vi "Shooter Wheel GetSet.vi"(9 "Enum":enum16{"Set", "Get"}(ring), 10 "Shooter Wheel DevRef In":T1={"Shooter Config reference"=refnum, "Shooter Data"={"MotorControlDevRef"={"DeviceStatus"={"status"=FALSE, "code"=0, "source"=""}, "Type"=enum."PWM", "PWM"={"PWM Channel"=enum."Invalid", "DeadBand"={"Name"="", "maxPositivePwm"=0, "minPositivePwm"=0, "centerPwm"=0, "maxNegativePwm"=0, "minNegativePwm"=0, "angularRange"=0}}, "CAN"={"Device Number"=0, "SetOutput VI Ref"=variant(enum8{"Percent VBus", "Current", "Speed", "Position", "Voltage"} enum."Percent VBus"), "GetOutput VI Ref"=variant(refnum<k1> refnum), "Enable VI Ref"=variant(dbl 12.0), "Disable VI Ref"=variant(enum8{"Percent VBus", "Speed", "Position", "Slave", "Unchanged / Invalid", "Voltage Compensation", "Current", "Motion Profile"} enum."Percent VBus"), "Data"=variant}, "Invert"=FALSE}, "CounterDevRef in"={"DevStatus"={"status"=FALSE, "code"=0, "source"=""}, "CntIndex"=enum."Ctr 0"}, "RPM Desired"=refnum, "RPM Actual"=refnum}}, 11 "DevRef":string) -> (0 "Error Out":errorcluster, 3 "Shooter Wheel DevRef Out":T1={"Shooter Config reference"=refnum, "Shooter Data"={"MotorControlDevRef"={"DeviceStatus"={"status"=FALSE, "code"=0, "source"=""}, "Type"=enum."PWM", "PWM"={"PWM Channel"=enum."Invalid", "DeadBand"={"Name"="", "maxPositivePwm"=0, "minPositivePwm"=0, "centerPwm"=0, "maxNegativePwm"=0, "minNegativePwm"=0, "angularRange"=0}}, "CAN"={"Device Number"=0, "SetOutput VI Ref"=variant(enum8{"Percent VBus", "Current", "Speed", "Position", "Voltage"} enum."Percent VBus"), "GetOutput VI Ref"=variant(refnum<k1> refnum), "Enable VI Ref"=variant(dbl 12.0), "Disable VI Ref"=variant(enum8{"Percent VBus", "Speed", "Position", "Slave", "Unchanged / Invalid", "Voltage Compensation", "Current", "Motion Profile"} enum."Percent VBus"), "Data"=variant}, "Invert"=FALSE}, "CounterDevRef in"={"DevStatus"={"status"=FALSE, "code"=0, "source"=""}, "CntIndex"=enum."Ctr 0"}, "RPM Desired"=refnum, "RPM Actual"=refnum}})   [LabVIEW 2016, in "Shooter _Wheel.lvlib"]
doc: "Help by FRC Team 836 - The RoboBees\n\nThis VI can either set or get the control parameters of a shooter wheel depending on the users command."
uses:
  <userlib>/836-Libraries/Motion_Control/Shooter_Wheel/Shooter _Wheel.lvlib
  <vilib>/Rock Robotics/SystemInterfaces/Counter/FPGA_CounterCtrSystemIndex.ctl
  <vilib>/Rock Robotics/WPI/Counter/WPI_CounterDevRef.ctl
  <vilib>/Rock Robotics/SystemInterfaces/DIO/FPGA_DIOPWMChannel.ctl
  <vilib>/Rock Robotics/WPI/PWM/WPI_PWMDeadband.ctl
  <vilib>/Rock Robotics/WPI/MotorControl/WPI_MotorControlDeviceRef.ctl
  <userlib>/836-Libraries/Motion_Control/Shooter_Wheel/ShooterData.ctl
  <userlib>/836-Libraries/Motion_Control/Shooter_Wheel/ShooterConfig.ctl
  <userlib>/836-Libraries/Motion_Control/Shooter_Wheel/ShooterControl.ctl
  <vilib>/Rock Robotics/WPI/MotorControl/WPI_MotorControlType.ctl
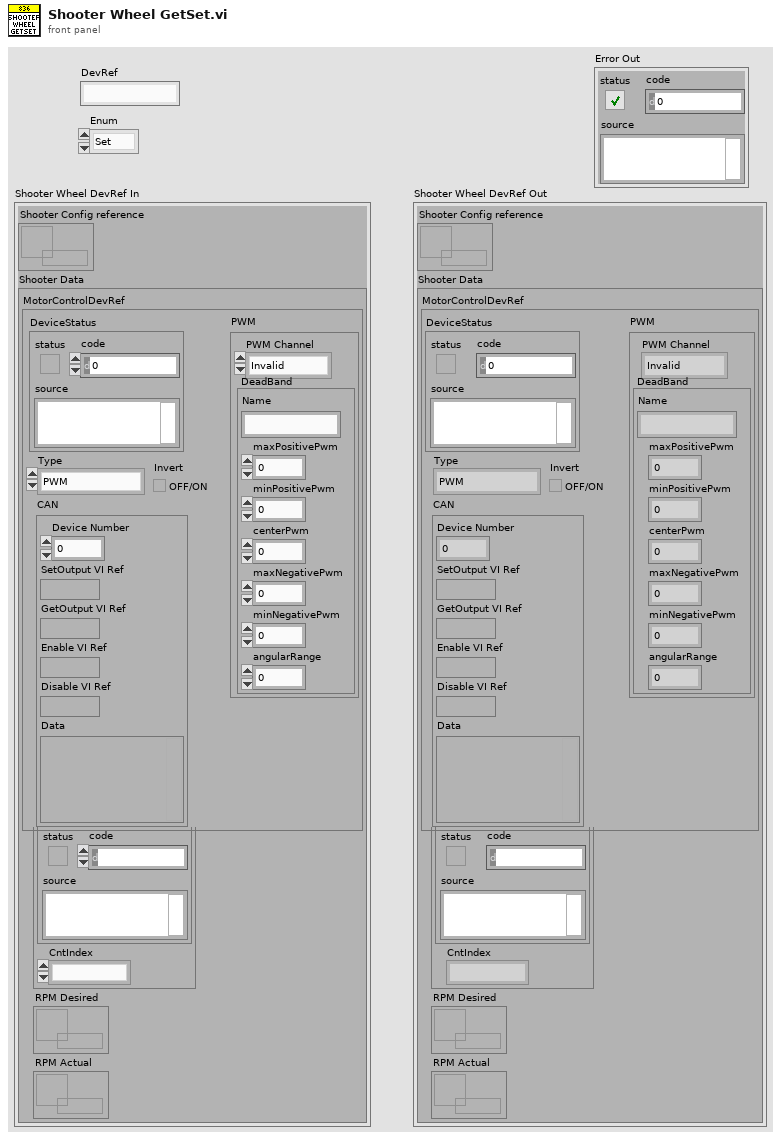
[diagram p1: front panel]
types:
  T1 = typedef "Shooter Wheel.lvlib/ShooterControl.ctl" = cluster{"Shooter Config reference":refnum<data-value>, "Shooter Data":T2}
  T2 = typedef "Shooter Wheel.lvlib/ShooterData.ctl" = cluster{"MotorControlDevRef":T3, "CounterDevRef in":T7, "RPM Desired":refnum<k33>, "RPM Actual":refnum<k33>}
  T3 = typedef "WPI_MotorControlDeviceRef.ctl" = cluster{"DeviceStatus":errorcluster, "Type":T4, "PWM":cluster{"PWM Channel":T5, "DeadBand":T6}, "CAN":cluster{"Device Number":u8, "SetOutput VI Ref":variant, "GetOutput VI Ref":variant, "Enable VI Ref":variant, "Disable VI Ref":variant, "Data":variant}, "Invert":bool}
  T4 = typedef "WPI_MotorControlType.ctl" = enum16{"PWM", "CAN"}
  T5 = typedef "FPGA_DIOPWMChannel.ctl" = enum8{"PWM 0", "PWM 1", "PWM 2", "PWM 3", "PWM 4", "PWM 5", "PWM 6", "PWM 7", "PWM 8", "PWM 9", "PWM MXP 0", "PWM MXP 1", "PWM MXP 2", "PWM MXP 3", "PWM MXP 4", "PWM MXP 5", "PWM MXP 6", "PWM MXP 7", "PWM MXP 8", "PWM MXP 9", "Invalid"}
  T6 = typedef "WPI_PWMDeadband.ctl" = cluster{"Name":string, "maxPositivePwm":i32, "minPositivePwm":i32, "centerPwm":i32, "maxNegativePwm":i32, "minNegativePwm":i32, "angularRange":u16}
  T7 = typedef "WPI_CounterDevRef.ctl" = cluster{"DevStatus":errorcluster, "CntIndex":T8}
  T8 = typedef "FPGA_CounterCtrSystemIndex.ctl" = enum8{"Ctr 0", "Ctr 1", "Ctr 2", "Ctr 3", "Ctr 4", "Ctr 5", "Ctr 6", "Ctr 7", "Invalid"}
  T9 = typedef "Shooter Wheel.lvlib/ShooterConfig.ctl" = cluster{"Period (ms)":i64, "TBH Gain":dbl, "Priority":i32}
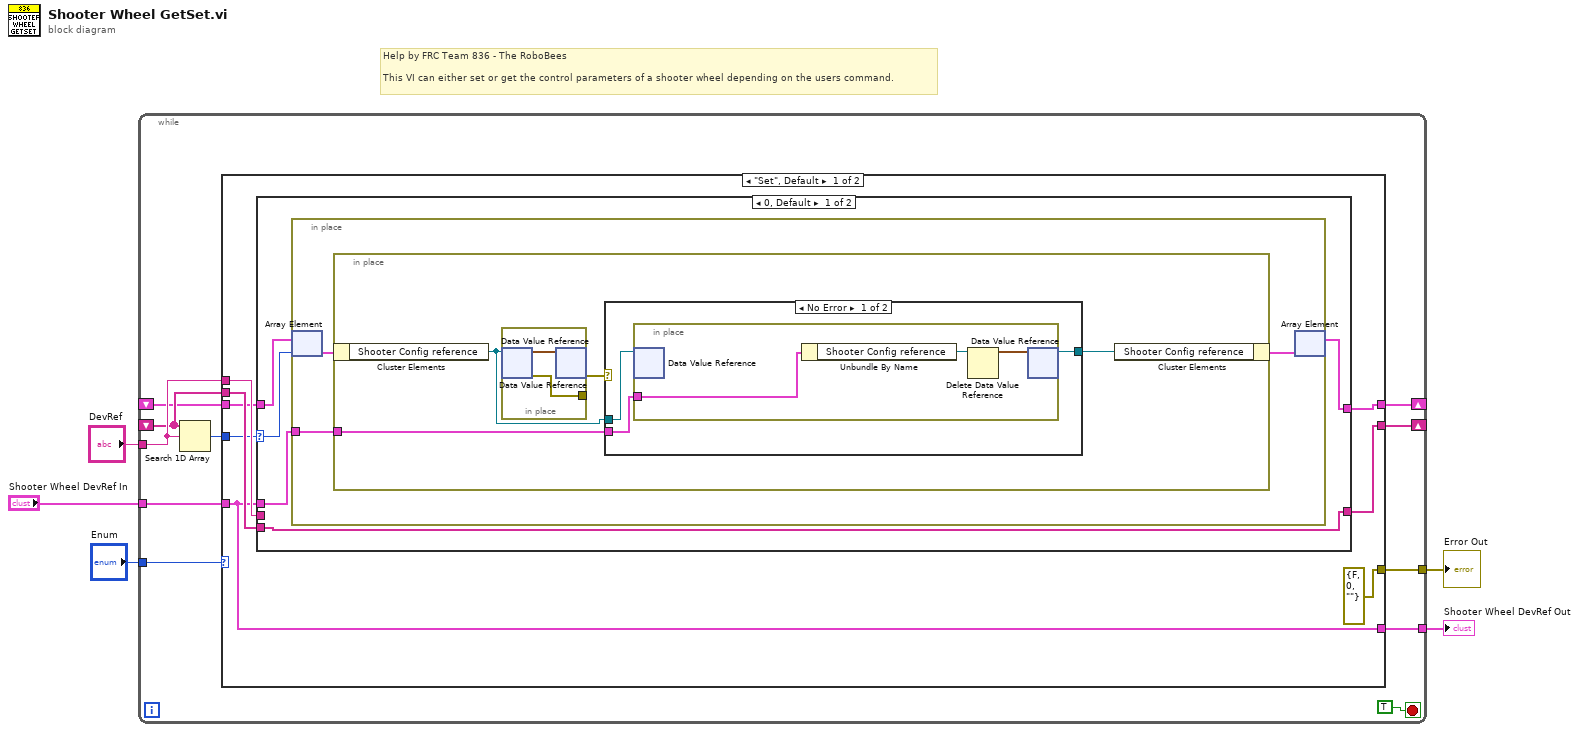
[diagram p0: block diagram]
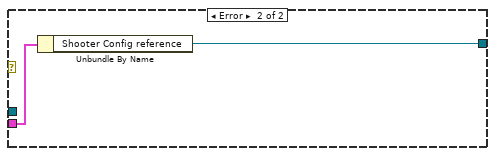
[diagram p2: hidden frame]
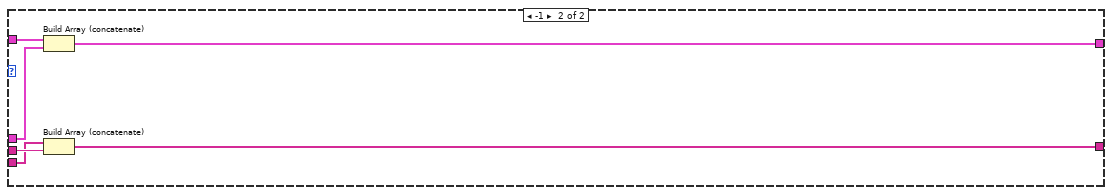
[diagram p3: hidden frame]
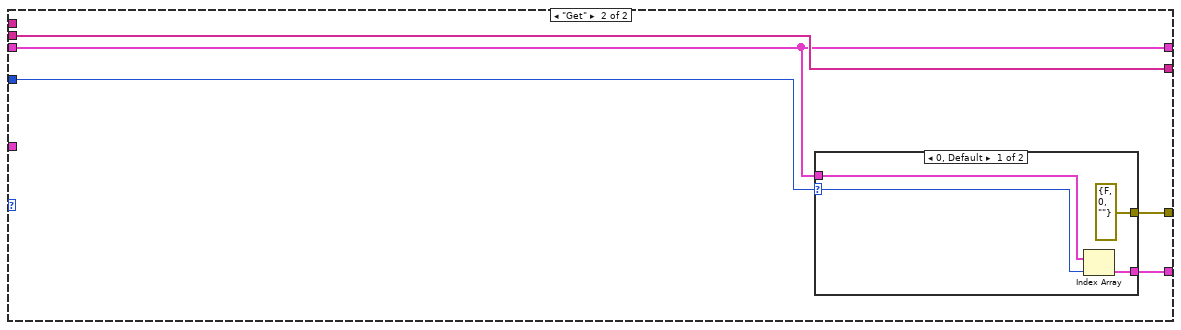
[diagram p4: hidden frame]
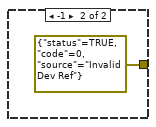
[diagram p5: hidden frame]
diagram:
  # "Help by FRC Team 836 - The RoboBees\n\nThis VI can either set or get the control parameters of a shooter wheel depending on the users command."
  n1 = while {
    shift-right: [w12] -> _
    shift-left: _ -> [w11]
    shift-right: [w15] -> _
    shift-left: _ -> [w14]
    tunnel: "DevRef" -> [w16]
    tunnel: "Shooter Wheel DevRef In" -> [w13]
    tunnel: [w8] -> w1
    tunnel: "Enum" -> [w7]
    tunnel: [w6] -> w3
    stop <- TRUE stop-if-true
    n2 = Search 1D Array(1D array=w14, element=w16) -> (index of element=w9:i32)  [unwired: 1 out]
    n3 = case shown="\"Set\", Default" w7 {
      tunnel: w16 -> [w24 _]
      tunnel: [w23 w57] -> w15
      tunnel: w14 -> [w22 w57]
      tunnel: w13 -> [w19 _]
      tunnel: [w21 w56] -> w12
      tunnel: w11 -> [w20 w56]
      tunnel: w9 -> [w17 w55]
      tunnel: [w19 w54] -> w8
      tunnel: [errorcluster {"status"=FALSE, "code"=0, "source"=""} ("error constant") w53] -> w6
      frame "Set", Default {
        n4 = case shown="0, Default" w17 {
          selector: w17 -> [w29 _]
          tunnel: [w25 w52] -> w21
          tunnel: [w28 w51] -> w23
          tunnel: w24 -> [_ w50]
          tunnel: w22 -> [w28 w49]
          tunnel: w19 -> [w26 w48]
          tunnel: w20 -> [w27 w47]
          frame 0, Default {
            n5 = in-place {
              in-place-border: w26 -> [w30]
              n6 = in-place-array #1(w27, w29) -> (w32:T1)
              n7 = in-place {
                in-place-border: w30 -> [w34]
                n8 = in-place-cluster #2(w32) -> ("Shooter Config reference"=w35:refnum<data-value>)
                n9 = in-place {
                  in-place-border: [w46] -> _
                  n10 = in-place-dvr #3(w35) -> (w45:T9, w46:errorcluster)
                  n11 = in-place-dvr #3(w45) -> (w33:errorcluster)  [unwired: 1 out]
                }
                n12 = case shown="No Error" w33 {
                  tunnel: [w39 w43] -> w36
                  tunnel: w34 -> [w38 w44]
                  tunnel: w35 -> [w37 _]
                  frame No Error {
                    n13 = in-place {
                      in-place-border: w38 -> [w42]
                      n14 = in-place-dvr #4(w37) -> ()  [unwired: 2 out]
                      n15 = Unbundle By Name(w42) -> ("Shooter Config reference"=w41:refnum<data-value>)
                      n16 = Delete Data Value Reference(data value reference=w41) -> (data value=w40:T9)  [unwired: 1 in, 1 out]
                      n17 = in-place-dvr #4(w40) -> (w39:refnum<data-value>)  [unwired: 1 out]
                    }
                  }
                  frame Error {
                    n18 = Unbundle By Name(w44) -> ("Shooter Config reference"=w43:refnum<data-value>)
                  }
                }
                n19 = in-place-cluster #2("Shooter Config reference"=w36) -> (w31:T1)
              }
              n20 = in-place-array #1(w31) -> (w25:T1[])  [unwired: 1 out]
            }
          }
          frame -1 {
            n21 = Build Array (concatenate)(w47, w48) -> (w52:T1[])
            n22 = Build Array (concatenate)(w49, w50) -> (w51:string[])
          }
        }
      }
      frame "Get" {
        n23 = case shown="0, Default" w55 {
          selector: w55 -> [w60 _]
          tunnel: w56 -> [w61 _]
          tunnel: [w59 _] -> w54
          tunnel: [errorcluster {"status"=FALSE, "code"=0, "source"=""} ("error constant") errorcluster {"status"=TRUE, "code"=0, "source"="Invalid Dev Ref"} ("error constant")] -> w53
          frame 0, Default {
            n24 = Index Array(array=w61, index=w60) -> (element=w59:T1)
          }
          frame -1 {
          }
        }
      }
    }
  }
  "Error Out" <- w3
  "Shooter Wheel DevRef Out" <- w1
